vi "Get Dynamic VI References.vi"(8 "error in (no error)":errorcluster, 11 "Channel Count":i32) -> (0 "error out":errorcluster, 3 "Dynamic VI References":refnum<vi>[](array[refnum]))   [LabVIEW 2013, in "Workspace MultiY Graph.lvlib"]
uses:
  Workspace MultiY Graph.lvlib
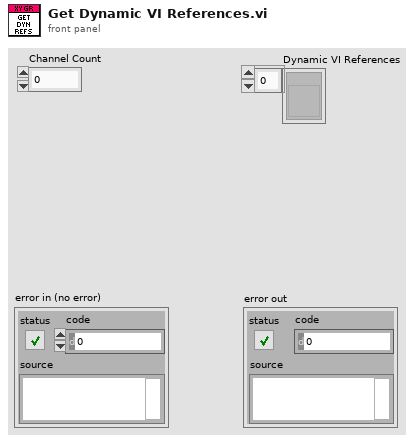
[diagram p1: front panel]
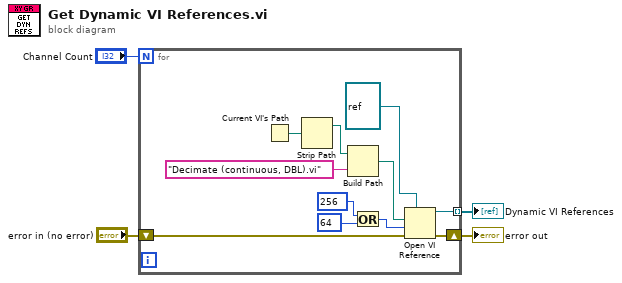
[diagram p0: block diagram]
diagram:
  n1 = for {
    N: "Channel Count" -> [_]
    tunnel: [w15] -> w4 mode=indexing
    shift-right: [w14] -> w3
    shift-left: "error in (no error)" -> [w6]
    n2 = Current VI's Path() -> (path=w12:path)
    n3 = Strip Path(path=w12) -> (stripped path=w5:path)  [unwired: 1 out]
    n4 = Build Path(base path=w5, name or relative path="Decimate (continuous, DBL).vi") -> (appended path=w11:path)
    n5 = Or(x=256 ("options"), y=64 ("options")) -> (x .or. y?=w7:i32)
    n6 = Open VI Reference(type specifier VI Refnum (for type only)=refnum<vi> refnum, vi path=w11, options=w7, error in (no error)=w6) -> (vi reference=w15:refnum<vi>, error out=w14:errorcluster)  [unwired: 2 in]
  }
  "Dynamic VI References" <- w4
  "error out" <- w3
